vi "Wait for reachability.vi"(7 "timeout (ms)":i32, 8 "error in (no error)":errorcluster, 10 "must be directly reachable?":bool, 11 "address":refnum<class "Generic Network Address.lvclass">) -> (0 "error out":errorcluster, 2 "found?":bool, 3 "address out":refnum<class "Generic Network Address.lvclass">)   [LabVIEW 2020, in "NI_WFCN.lvlib" / "Generic Network Address.lvclass"]
doc: "Waits until the local system can attempt to contact the specified host."
uses:
  <vilib>/net/WFCN/Addressing/Generic Network Address/Generic Network Address.lvclass
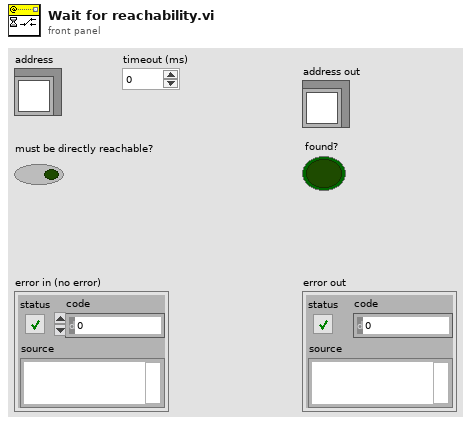
[diagram p1: front panel]
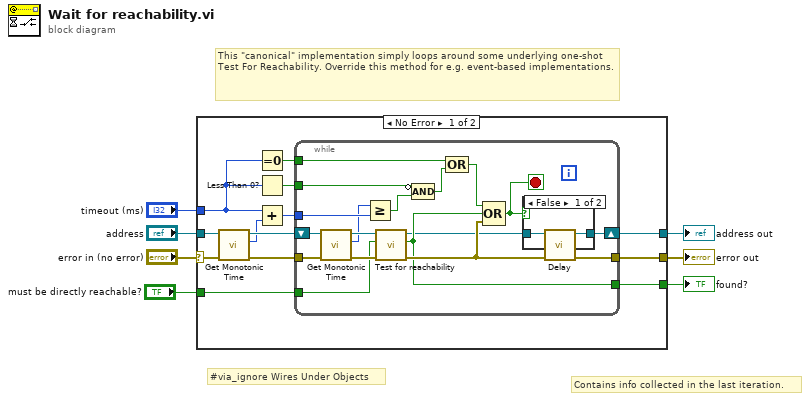
[diagram p0: block diagram]
diagram:
  # "#via_ignore Wires Under Objects"
  # "Contains info collected in the last iteration."
  # "This \"canonical\" implementation simply loops around some underlying one-shot Test For Reachability. Override this method for e.g. event-based implementations."
  n1 = case shown="No Error" "error in (no error)" {
    selector: "error in (no error)" -> [w9 w40]
    tunnel: [w19 w40] -> w7
    tunnel: "timeout (ms)" -> [w18 _]
    tunnel: "address" -> [w15 w39]
    tunnel: [w17 _] -> w4
    tunnel: [w16 w39] -> w3
    tunnel: "must be directly reachable?" -> [w8 _]
    frame No Error {
      n2 = call-dynamic "Get Monotonic Time.vi"("Generic Network Address in"=w15) -> ("timestamp"=w10:u32, "Generic Network Address out"=w11:refnum<class "Generic Network Address.lvclass">)  [unwired: 9 in]
      n3 = Equal To 0?(x=w18) -> (x = 0?=w12:bool)
      n4 = Less Than 0?(x=w18) -> (x < 0?=w14:bool)
      n5 = Add(x=w18, y=w10) -> (x+y=w13:u32)
      n6 = while {
        tunnel: w13 -> [w35]
        tunnel: w14 -> [w27]
        tunnel: [w32] -> w17
        shift-right: [w29] -> w16
        shift-left: w11 -> [w23]
        tunnel: w12 -> [w28]
        tunnel: [w34] -> w19
        tunnel: w9 -> [w21]
        tunnel: w8 -> [w20]
        stop <- w33 stop-if-true
        n7 = call-dynamic "Get Monotonic Time.vi"("Generic Network Address in"=w23) -> ("timestamp"=w22:u32, "Generic Network Address out"=w31:refnum<class "Generic Network Address.lvclass">)  [unwired: 9 in]
        n8 = Greater Or Equal?(x=w22, y=w35) -> (x >= y?=w25:bool)
        n9 = call-dynamic "Test for reachability.vi"("error in (no error)"=w21, "must be directly reachable?"=w20, "address"=w31) -> ("error out"=w34:errorcluster, "found?"=w32:bool, "address out"=w30:refnum<class "Generic Network Address.lvclass">)  [unwired: 6 in]
        n10 = Compound Arithmetic op=AND(invert w27, w25) -> (w26:bool)
        n11 = Compound Arithmetic op=OR(w28, w26) -> (w24:bool)
        n12 = Compound Arithmetic op=OR(w24, w32, w34) -> (w33:bool)
        n13 = case shown="False" w33 {
          tunnel: w30 -> [w37 w38]
          tunnel: [w36 w38] -> w29
          frame False {
            n14 = call-dynamic "Delay.vi"("address"=w37) -> ("address out"=w36:refnum<class "Generic Network Address.lvclass">)  [unwired: 10 in]
          }
          frame True {
          }
        }
      }
    }
    frame Error {
    }
  }
  "error out" <- w7
  "found?" <- w4
  "address out" <- w3
